vi "Configure Output Adjustment.vi"(7 "Adjustment Direction (0: Increment)":i32(ring) items=["Increment", "Decrement"], 8 "error in (no error)":errorcluster, 9 "Adjustment Value (0)":dbl, 10 "Adjustment Type (0: Multiply)":i32(ring) items=["Multiply", "Increments or Decrements"], 11 "VISA resource name":refnum<visa-resource-name>) -> (0 "error out":errorcluster, 3 "VISA resource name out":refnum<visa-resource-name>)   [LabVIEW 2012, in "Fluke 5080.lvlib"]
doc: "Supplies the adjustment methods for calibration output value."
uses:
  <instrlib>/Fluke 5080/Fluke 5080.lvlib
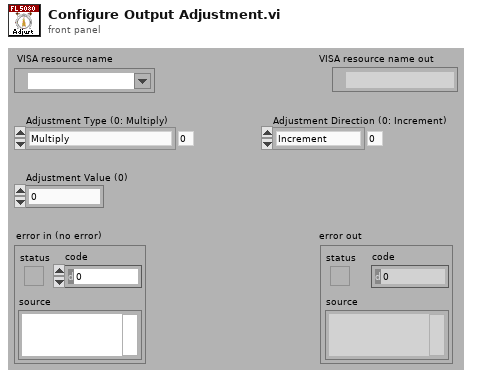
[diagram p1: front panel]
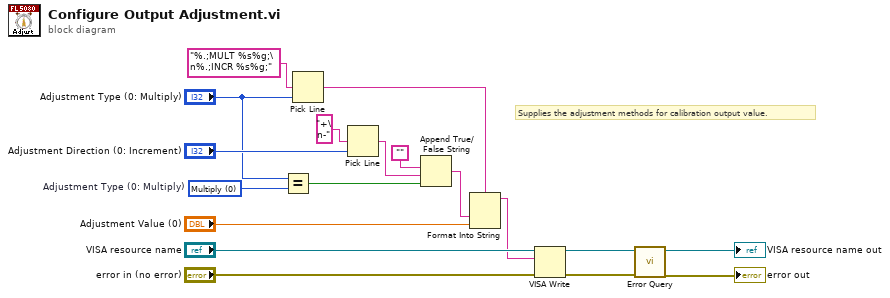
[diagram p0: block diagram]
diagram:
  w3 = 0 items=["Multiply", "Increments or Decrements"]  # Adjustment Type (0: Multiply)
  # "Supplies the adjustment methods for calibration output value."
  n1 = Equal?(x="Adjustment Type (0: Multiply)", y=w3) -> (x = y?=w2:bool)
  n2 = Pick Line(multi-line string="%.;MULT %s%g;\n%.;INCR %s%g;", line index="Adjustment Type (0: Multiply)") -> (output string=w10:string)  [unwired: 1 out]
  n3 = Pick Line(multi-line string="+\n-", line index="Adjustment Direction (0: Increment)") -> (output string=w6:string)  [unwired: 1 out]
  n4 = Append True/False String(1:w2, 2:w6, 3:"") -> (0:w7:string)  [unwired: 1 out]
  n5 = Format Into String(format string=w10, w7, "Adjustment Value (0)") -> (resulting string=w1:string)  [unwired: 2 in, 1 out]
  n6 = VISA Write(VISA resource name="VISA resource name", write buffer=w1, error in (no error)="error in (no error)") -> (VISA resource name out=w16:refnum<visa-resource-name>, error out=w15:errorcluster)  [unwired: 1 out]
  n7 = call <instrlib>:"Error Query.vi"("error in (no error)"=w15, "VISA resource name"=w16) -> ("error out"=→"error out":errorcluster, "VISA resource name out"=→"VISA resource name out":refnum<visa-resource-name>)  [unwired: 8 out]
